vi "Read_OPC_Product_Counter.vi"(4 "Counter":u32[](array[numeric])) -> (0 "Counter_Number":i32, 2 "Counter_String":string)   [LabVIEW 2017]
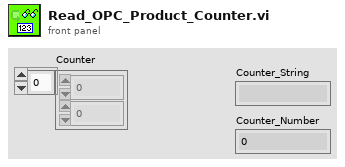
[diagram p1: front panel]
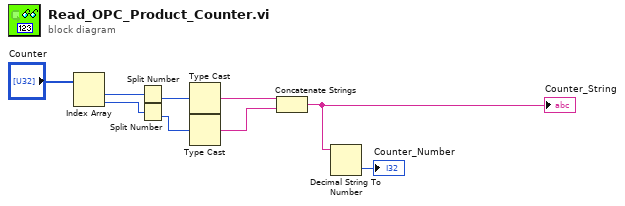
[diagram p0: block diagram]
diagram:
  n1 = Index Array(array="Counter") -> (element #1=w4:u32, element #2=w2:u32)  [unwired: 2 in]
  n2 = Split Number(x=w4) -> (lo(x)=w3:u16)  [unwired: 1 out]
  n3 = Split Number(x=w2) -> (lo(x)=w1:u16)  [unwired: 1 out]
  n4 = Type Cast(x=w3) -> (*(type *) &x=w8:string)  [unwired: 1 in]
  n5 = Type Cast(x=w1) -> (*(type *) &x=w7:string)  [unwired: 1 in]
  n6 = Concatenate Strings(w8, w7) -> (w6:string)
  "Counter_String" <- w6
  n7 = Decimal String To Number(string=w6) -> (number=→"Counter_Number":i32)  [unwired: 2 in, 1 out]
